vi "LPF.vi"(11 "Subset 3":dbl[](array[numeric])) -> (3 "Filtered X":dbl[](array[numeric]))   [LabVIEW 2018]
uses:
  <vilib>/Analysis/NI_AALBase.lvlib
  <vilib>/Analysis/3filter.llb/Butterworth Filter (DBL).vi
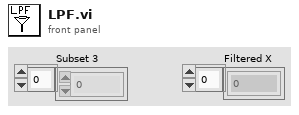
[diagram p1: front panel]
types:
  T1 = enum16{"Lowpass", "Highpass", "Bandpass", "Bandstop"}
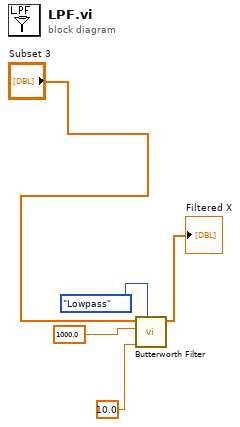
[diagram p0: block diagram]
diagram:
  n1 = call-poly <vilib>:"Butterworth Filter.vi"("filter type"=T1."Lowpass", "low cutoff freq: fl"=10.0, "sampling freq: fs"=1000.0, "X"="Subset 3") -> ("Filtered X"=→"Filtered X":dbl[])  [unwired: 4 in, 1 out]
